vi "Get State.vi"(8 "error in (no error)":errorcluster, 11 "Pulse Controller in":refnum<class "Channel Scanner.lvclass">) -> (0 "error out":errorcluster, 1 "Result ready":bool, 2 "Armed":bool, 3 "Pulse Controller out":refnum<class "Channel Scanner.lvclass">, 4 "Check again":bool)   [LabVIEW 2019, in "Channel Scanner.lvclass"]
uses:
  Channel Scanner.lvclass
  Channel Scanner.lvclass/Channel Scanner.ctl
  Instrument Actor/Instrument Actor.lvclass
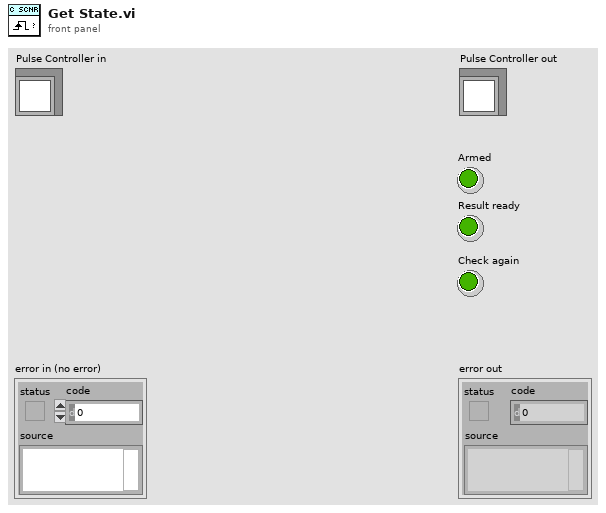
[diagram p1: front panel]
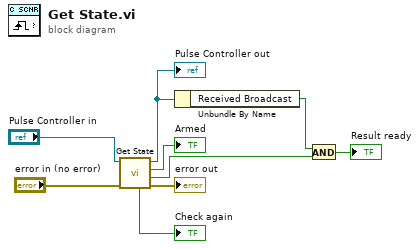
[diagram p0: block diagram]
diagram:
  n1 = call-parent "Get State.vi"("error in (no error)"="error in (no error)", "Instrument Actor in"="Pulse Controller in") -> ("error out"=→"error out":errorcluster, "Result ready"=w4:bool, "Armed"=→"Armed":bool, "Instrument Actor out"=w5:refnum<class "Channel Scanner.lvclass">, "Check again"=→"Check again":bool)  [unwired: 5 in]
  "Pulse Controller out" <- w5
  n2 = Unbundle By Name(w5) -> ("Received Broadcast"=w3:bool)
  n3 = And(x=w3, y=w4) -> (x .and. y?=→"Result ready":bool)
